vi "Async Get averaged image from CamServer.vi"(4 "Quality":u32=750 max=1000, 6 "Resolution":T1 items=["Low", "Med.", "High", "Max."], 7 "Camera":T2="Travcam", 8 "Averaging time (s) (from end)":dbl=1.0 format="%#_13g", 9 "Duration (s)":dbl=10.0 format="%#_13g", 10 "Image name":string="test", 11 "Image directory path":path=path "C:/test") -> (0 "Error out":errorcluster, 3 "Image file path":path)   [LabVIEW 2015]
doc: "Asynchronously gets a time-averaged image from the selected camera on the camera server and saves it to the specified path with specified name.s"
uses:
  Camera enum/Camera enum.ctl
  Camera enum/Camera resolution.ctl
  Globals/CamServer global.vi
panel:
  # "PN 21/08/15"
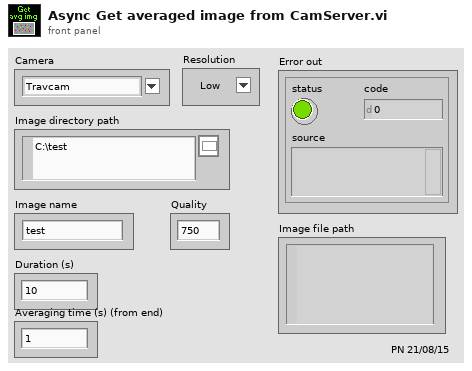
[diagram p1: front panel]
types:
  T1 = typedef "Camera resolution.ctl" = u8
  T2 = typedef "Camera enum.ctl" = string
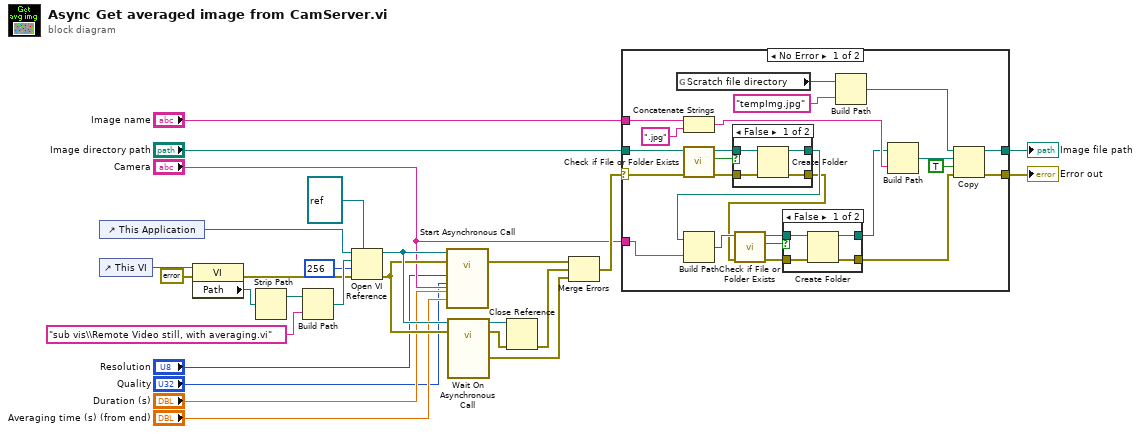
[diagram p0: block diagram]
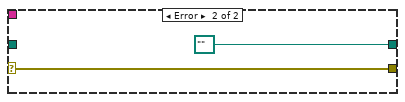
[diagram p4: hidden frame]
diagram:
  n1 = control-ref of="This Application"() -> (w22:refnum<vi>)
  n2 = control-ref of="This VI"() -> (w27:refnum<vi>)
  n3 = property class="VI"(reference=w27, error in=errorcluster {"status"=FALSE, "code"=0, "source"=""} ("error in (no error)")) -> (error out=w24:errorcluster, "Path"=w20:path)  [unwired: 1 out]
  n4 = Strip Path(path=w20) -> (stripped path=w19:path)  [unwired: 1 out]
  n5 = Build Path(base path=w19, name or relative path="sub vis\\Remote Video still, with averaging.vi") -> (appended path=w25:path)
  n6 = Open VI Reference(type specifier VI Refnum (for type only)=refnum<vi> refnum, application reference (local)=w22, vi path=w25, options=256, error in (no error)=w24) -> (vi reference=w18:refnum<vi>, error out=w17:errorcluster)  [unwired: 1 in]
  n7 = call-by-ref "Start Asynchronous Call"(reference=w18, error in=w17, "Resolution"="Resolution", "Quality"="Quality", "Duration (s)"="Duration (s)", "Averaging time (s) (from end)"="Averaging time (s) (from end)", "Camera"="Camera") -> (error out=w15:errorcluster)  [unwired: 2 out]
  n8 = call-by-ref "Wait On Asynchronous Call"(reference=w18, error in=w17) -> (reference out=w16:refnum<vi>, error out=w14:errorcluster, "Error out"=w12:errorcluster)  [unwired: 5 in]
  n9 = Close Reference(reference=w16, error in (no error)=w14) -> (error out=w13:errorcluster)
  n10 = Merge Errors(w15, w13, w12) -> (w5:errorcluster)
  n11 = case shown="No Error" w5 {
    selector: w5 -> [w50 w65]
    tunnel: "Image directory path" -> [w51 _]
    tunnel: "Image name" -> [w45 _]
    tunnel: [w29 w65] -> w8
    tunnel: "Camera" -> [w34 _]
    tunnel: [w28 path "" ("new path")] -> w3
    frame No Error {
      n12 = global read "CamServer global.vi" "Scratch file directory"() -> (w40:path)
      n13 = Concatenate Strings(w45, ".jpg" ("string")) -> (w43:string)
      n14 = call <vilib>:"Check if File or Folder Exists.vi"("error in (no error)"=w50, "path"=w51) -> ("error out"=w47:errorcluster, "file or folder exists?"=w49:bool, "dup path"=w48:path)  [unwired: 7 in]
      n15 = case shown="False" w49 {
        tunnel: w48 -> [w61 w63]
        tunnel: w47 -> [w60 w62]
        tunnel: [w59 w63] -> w35
        tunnel: [w58 w62] -> w32
        frame False {
          n16 = Create Folder(path (use dialog)=w61, error in=w60) -> (created path=w59:path, error out=w58:errorcluster)  [unwired: 1 in, 1 out]
        }
        frame True {
        }
      }
      n17 = Build Path(base path=w35, name or relative path=w34) -> (appended path=w33:path)
      n18 = call <vilib>:"Check if File or Folder Exists.vi"("error in (no error)"=w32, "path"=w33) -> ("error out"=w36:errorcluster, "file or folder exists?"=w37:bool, "dup path"=w38:path)  [unwired: 7 in]
      n19 = case shown="False" w37 {
        tunnel: w38 -> [w55 w57]
        tunnel: w36 -> [w54 w56]
        tunnel: [w53 w57] -> w31
        tunnel: [w52 w56] -> w30
        frame False {
          n20 = Create Folder(path (use dialog)=w55, error in=w54) -> (created path=w53:path, error out=w52:errorcluster)  [unwired: 1 in, 1 out]
        }
        frame True {
        }
      }
      n21 = Build Path(base path=w40, name or relative path="tempImg.jpg") -> (appended path=w39:path)
      n22 = Build Path(base path=w31, name or relative path=w43) -> (appended path=w44:path)
      n23 = Copy(8:w30, 9:TRUE ("overwrite (F)"), 10:w44, 11:w39) -> (0:w29:errorcluster, 3:w28:path)  [unwired: 1 in, 1 out]
    }
    frame Error {
    }
  }
  "Error out" <- w8
  "Image file path" <- w3
